vi "solar_misc Edit Help Link.vi"() -> ()   [LabVIEW 2018]
doc: "This VI exports a folder of VIs connector pane images to the output directory."
panel:
  in  "Add #Page Links? (F)":bool
  in  "Help Webpage":string
  in  "Folders to Exclude":string[](array[string])=["_builds", "_dev", "_vipb", "_vip"]
  in  "error in (no error)":errorcluster
  out "error out":errorcluster
  out "Complete":dbl(slide) scale=0.0..100.0
  in  "RootDir":path=path "C:/Projects/solar/LV2016/solar"
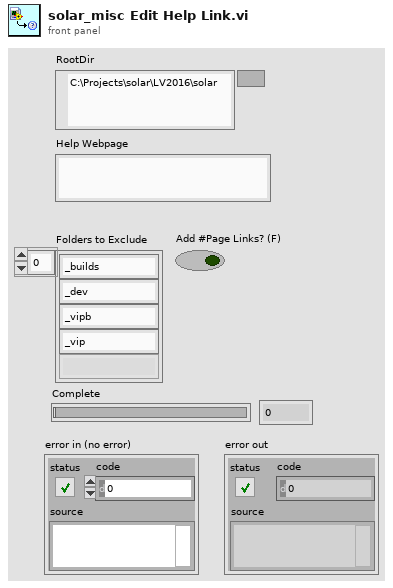
[diagram p1: front panel]
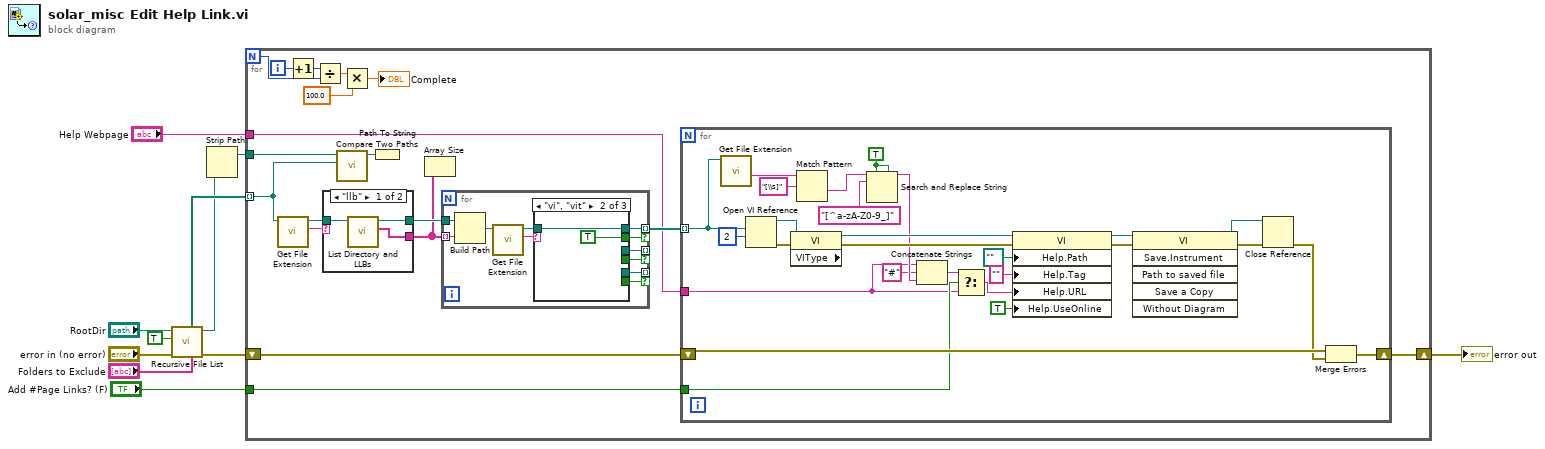
[diagram p0: block diagram]
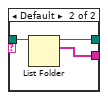
[diagram p2: hidden frame]
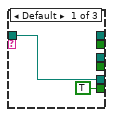
[diagram p3: hidden frame]
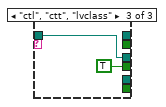
[diagram p4: hidden frame]
diagram:
  n1 = call <vilib>:"Recursive File List.vi"("Folders to Exclude"="Folders to Exclude", "error in (no error)"="error in (no error)", "Treat LLBs as Folders?"=TRUE, "Folder Path"="RootDir") -> ("error out"=w3:errorcluster, "dup Folder Path"=w7:path, "All Folders"=w10:path[])  [unwired: 3 in, 2 out]
  n2 = Strip Path(path=w7) -> (stripped path=w8:path)  [unwired: 1 out]
  n3 = for {
    N -> [w22]
    tunnel: w10 -> [w26] mode=indexing
    tunnel: w8 -> [w25]
    shift-right: [w15] -> w4
    shift-left: w3 -> [w14]
    tunnel: "Help Webpage" -> [w13]
    tunnel: "Add #Page Links? (F)" -> [w12]
    i -> [w23]
    n4 = call <vilib>:"Get File Extension.vi"("file"=w26) -> ("lowercase file extension"=w28:string, "dup file"=w27:path)  [unwired: 6 in, 3 out]
    n5 = Increment(x=w23) -> (x+1=w21:i32)
    n6 = Divide(x=w21, y=w22) -> (x/y=w20:dbl)
    n7 = case shown="\"llb\"" w28 {
      tunnel: w27 -> [w32 w35]
      tunnel: [w31 w34] -> w29
      tunnel: [w30 w33] -> w24
      frame "llb" {
        n8 = call <vilib>:"List Directory and LLBs.vi"("Folder Path"=w32) -> ("Files sans LLBs"=w30:string[], "dup Folder Path"=w31:path)  [unwired: 2 in, 7 out]
      }
      frame Default {
        n9 = List Folder(path=w35) -> (path out=w34:path, filenames=w33:string[])  [unwired: 3 in, 2 out]
      }
    }
    n10 = call <vilib>:"Compare Two Paths.vi"("Path 2"=w26, "Path 1"=w25) -> ("Relative Path from 1 to 2"=w17:path)  [unwired: 6 in, 3 out]
    n11 = Multiply(x=w20, y=100.0) -> (x*y=→"Complete":dbl)
    n12 = Path To String(path=w17) -> ()  [unwired: 1 out]
    n13 = Array Size(array=w24) -> ()  [unwired: 1 out]
    n14 = for {
      tunnel: w29 -> [w46]
      tunnel: w24 -> [w45] mode=indexing
      tunnel: [w42] -> w16 mode=indexing if=w38
      tunnel: [w40] -> _ mode=indexing if=w39
      tunnel: [w37] -> _ mode=indexing if=w36
      n15 = Build Path(base path=w46, name or relative path=w45) -> (appended path=w44:path)
      n16 = call <vilib>:"Get File Extension.vi"("file"=w44) -> ("lowercase file extension"=w43:string, "dup file"=w41:path)  [unwired: 6 in, 3 out]
      n17 = case shown="\"vi\", \"vit\"" w43 {
        tunnel: [_ w50 _] -> w42
        tunnel: w41 -> [w48 w50 w51]
        tunnel: [_ _ w51] -> w40
        tunnel: [_ _ TRUE] -> w39
        tunnel: [_ TRUE _] -> w38
        tunnel: [w48 _ _] -> w37
        tunnel: [TRUE _ _] -> w36
        frame Default {
        }
        frame "vi", "vit" {
        }
        frame "ctl", "ctt", "lvclass" {
        }
      }
    }
    n18 = for {
      tunnel: w16 -> [w64] mode=indexing
      shift-right: [w79] -> w15
      shift-left: w14 -> [w78]
      tunnel: w13 -> [w54]
      tunnel: w12 -> [w55]
      w60 = TRUE ("replace all?")
      n19 = call <vilib>:"Get File Extension.vi"("file"=w64) -> ("filename without extension"=w63:string)  [unwired: 6 in, 4 out]
      n20 = Open VI Reference(vi path=w64, options=2) -> (vi reference=w67:refnum<vi>, error out=w77:errorcluster)  [unwired: 4 in]
      n21 = property class="VI" props=["VIType"](reference=w67, error in=w77) -> (reference out=w66:refnum<vi>, error out=w68:errorcluster)  [unwired: 1 out]
      n22 = Match Pattern(string=w63, regular expression="[\\s]") -> (after substring=w59:string)  [unwired: 1 in, 3 out]
      n23 = Search and Replace String(replace all?=w60, multiline?=w60, input string=w59, search string="[^a-zA-Z0-9_]") -> (result string=w58:string)  [unwired: 4 in, 3 out]
      n24 = Concatenate Strings(w54, "#" ("string"), w58) -> (w56:string)
      n25 = Select(t=w56, s=w55, f=w54) -> (s? t:f=w53:string)
      n26 = property class="VI"(reference=w66, error in=w68, "Help.Path"=path "" ("Help:Document Path"), "Help.Tag"="" ("Help:Document Tag"), "Help.URL"=w53, "Help.UseOnline"=TRUE ("Help:Use Web URL")) -> (reference out=w74:refnum<vi>, error out=w76:errorcluster)
      n27 = invoke class="VI" method="Save.Instrument"(reference=w74, error in=w76) -> (reference out=w73:refnum<vi>, error out=w75:errorcluster)  [unwired: 4 in, 4 out]
      n28 = Close Reference(reference=w73, error in (no error)=w75) -> (error out=w72:errorcluster)
      n29 = Merge Errors(w78, w72) -> (w79:errorcluster)
    }
  }
  "error out" <- w4
